vi "MoveAbs.vi"(8 "error in (no error)":errorcluster, 11 "ZanClass in":refnum<class "ZanClass.lvclass">) -> (0 "error out":errorcluster, 3 "ZanClass out":refnum<class "ZanClass.lvclass">)   [LabVIEW 2019, in "ZanClass.lvclass"]
uses:
  ZanClass.lvclass
  LLB/zmotion/zaux/zauxdll.lvlib
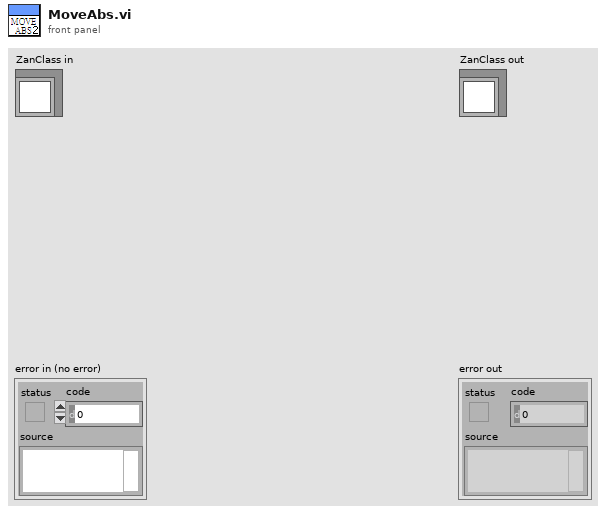
[diagram p1: front panel]
types:
  T1 = cluster{"AxisName":string, "Accel":dbl, "Deaccel":dbl, "Speed":dbl, "Sramp":dbl}[]
  T2 = typedef "IO Card_Type.ctl" = enum16{"None", "Unidaq32", "6480", "2410C-64", "Zan", "DMC1000B", "16InOut", "Robot", "DMC3600"}
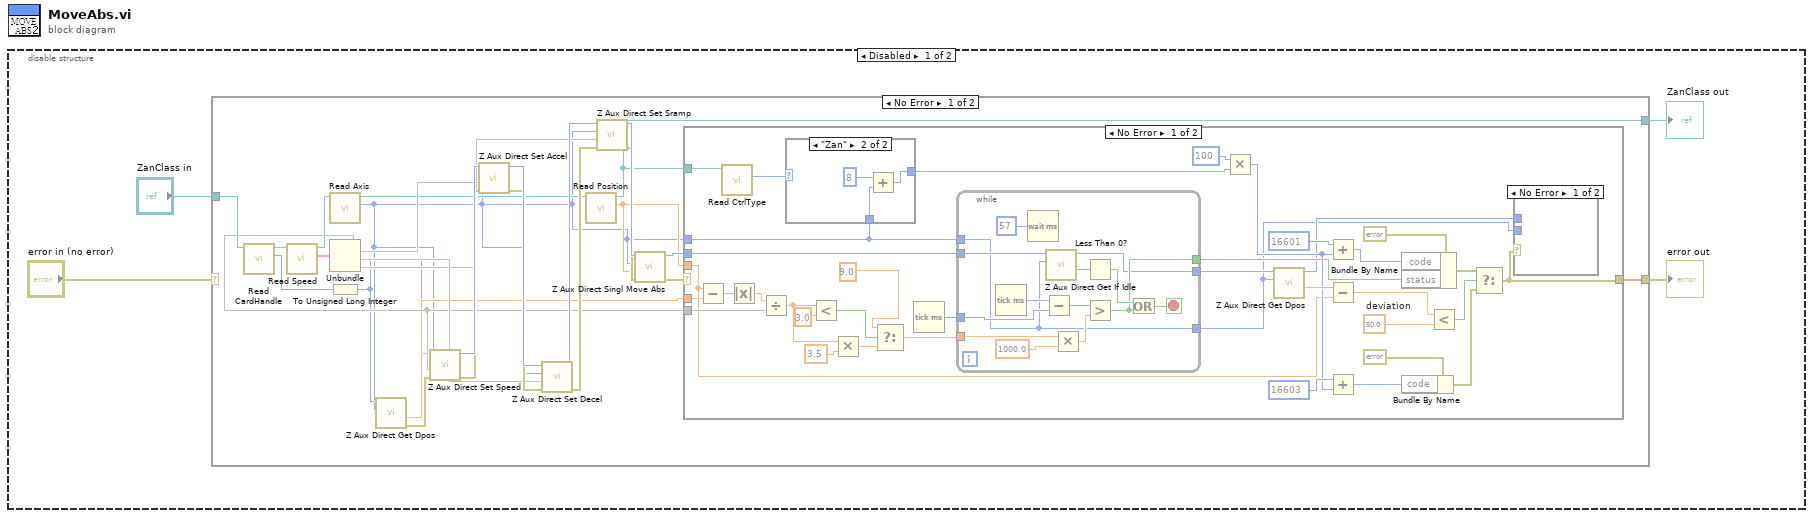
[diagram p0: block diagram]
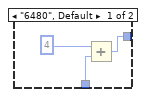
[diagram p2: hidden frame]
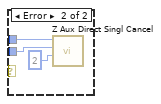
[diagram p3: hidden frame]
diagram:
  n1 = disable-structure shown="Disabled" {
    frame Disabled {
      n2 = case shown="No Error" "error in (no error)" {
        selector: "error in (no error)" -> [_ w93]
        tunnel: "ZanClass in" -> [w31 w94]
        tunnel: [w10 w93] -> w1
        tunnel: [w5 w94] -> w2
        frame No Error {
          n3 = call-dynamic "Read CardHandle.vi"("AxisCard in"=w31) -> ("CardHandle"=w30:i32, "AxisCard out"=w26:refnum<class "ZanClass.lvclass">)  [unwired: 8 in, 1 out]
          n4 = call-dynamic "Read Speed.vi"("AxisCard in"=w26) -> ("AxisSpeed"=w24:T1, "AxisCard out"=w25:refnum<class "ZanClass.lvclass">)  [unwired: 8 in, 1 out]
          n5 = call-dynamic "Read Axis.vi"("AxisCard in"=w25) -> ("Axis"=w6:u32, "AxisCard out"=w16:refnum<class "ZanClass.lvclass">)  [unwired: 8 in, 1 out]
          n6 = Unbundle(w24) -> (w12, w23, w19, w18)
          n7 = To Unsigned Long Integer(number=w30) -> (unsigned 32bit integer=w7:u32)
          n8 = call "Z Aux Direct Get Dpos.vi"("iaxis"=w6, "handle"=w7) -> ("error out"=w8:errorcluster, "pfValue out"=w9:sgl)  [unwired: 6 in, 2 out]
          n9 = call "Z Aux Direct Set Speed.vi"("error in (no error)"=w8, "fValue"=w12, "iaxis"=w6, "handle"=w7) -> ("error out"=w22:errorcluster, "handle out"=w29:u32)  [unwired: 5 in, 1 out]
          n10 = call "Z Aux Direct Set Accel.vi"("error in (no error)"=w22, "fValue"=w23, "iaxis"=w6, "handle"=w29) -> ("error out"=w21:errorcluster, "handle out"=w28:u32)  [unwired: 5 in, 1 out]
          n11 = call "Z Aux Direct Set Decel.vi"("error in (no error)"=w21, "fValue"=w19, "iaxis"=w6, "handle"=w28) -> ("error out"=w20:errorcluster, "handle out"=w27:u32)  [unwired: 5 in, 1 out]
          n12 = call-dynamic "Read Position.vi"("AxisCard in"=w16) -> ("Position"=w11:dbl, "AxisCard out"=w5:refnum<class "ZanClass.lvclass">)  [unwired: 8 in, 1 out]
          n13 = call "Z Aux Direct Set Sramp.vi"("error in (no error)"=w20, "fValue"=w18, "iaxis"=w6, "handle"=w27) -> ("error out"=w15:errorcluster, "handle out"=w17:u32)  [unwired: 5 in, 1 out]
          n14 = call "Z Aux Direct Singl Move Abs.vi"("error in (no error)"=w15, "fdistance"=w11, "iaxis"=w6, "handle"=w17) -> ("error out"=w14:errorcluster, "handle out"=w13:u32)  [unwired: 5 in, 1 out]
          n15 = case shown="No Error" w14 {
            selector: w14 -> [_ w92]
            tunnel: w13 -> [w68 _]
            tunnel: w6 -> [w35 _]
            tunnel: w12 -> [w46 _]
            tunnel: w11 -> [w40 _]
            tunnel: [w50 w92] -> w10
            tunnel: w9 -> [w39 _]
            tunnel: w5 -> [w38 _]
            frame No Error {
              w60 = 50.0  # deviation
              n16 = Subtract(x=w40, y=w39) -> (x-y=w42:dbl)
              n17 = call-dynamic "Read CtrlType.vi"("AxisCard in"=w38) -> ("IO Card Type"=w37:T2)  [unwired: 8 in, 2 out]
              n18 = Absolute Value(x=w42) -> (abs(x)=w41:dbl)
              n19 = Divide(x=w41, y=w46) -> (x/y=w33:dbl)
              n20 = case shown="\"Zan\"" w37 {
                tunnel: [w71 w74] -> w36
                tunnel: w35 -> [w69 w72]
                frame "6480", Default {
                  n21 = Add(x=4, y=w69) -> (x+y=w71:u32)
                }
                frame "Zan" {
                  n22 = Add(x=8, y=w72) -> (x+y=w74:u32)
                }
              }
              n23 = Less?(x=w33, y=3.0) -> (x < y?=w45:bool)
              n24 = Multiply(x=w33, y=3.5) -> (x*y=w44:dbl)
              n25 = Select(t=9.0, s=w45, f=w44) -> (s? t:f=w43:dbl)
              n26 = Tick Count (ms)() -> (millisecond timer value=w67:u32)
              n27 = while {
                tunnel: w68 -> [w91]
                tunnel: w35 -> [w79]
                tunnel: w67 -> [w86]
                tunnel: [w81] -> w54
                tunnel: [w80] -> w63
                tunnel: [w79] -> w48
                tunnel: w43 -> [w78]
                stop <- w82 stop-if-true
                n28 = Tick Count (ms)() -> (millisecond timer value=w87:u32)
                n29 = Wait (ms)(milliseconds to wait=u32 57) -> ()  [unwired: 1 out]
                n30 = Subtract(x=w87, y=w86) -> (x-y=w85:u32)
                n31 = call "Z Aux Direct Get If Idle.vi"("iaxis"=w79, "handle"=w91) -> ("piValue out"=w90:i32, "handle out"=w80:u32)  [unwired: 6 in, 2 out]
                n32 = Multiply(x=w78, y=1000.0) -> (x*y=w84:dbl)
                n33 = Less Than 0?(x=w90) -> (x < 0?=w83:bool)
                n34 = Greater?(x=w85, y=w84) -> (0:w81:bool)
                n35 = Or(x=w83, y=w81) -> (x .or. y?=w82:bool)
              }
              n36 = Multiply(x=u32 100, y=w36) -> (x*y=w58:u32)
              n37 = call "Z Aux Direct Get Dpos.vi"("iaxis"=w48, "handle"=w63) -> ("pfValue out"=w62:sgl, "handle out"=w49:u32)  [unwired: 6 in, 2 out]
              n38 = Add(x=16601 ("code"), y=w58) -> (x+y=w65:u32)
              n39 = Subtract(x=w62, y=w40) -> (x-y=w61:dbl)
              n40 = Add(x=16603 ("code"), y=w58) -> (x+y=w56:u32)
              n41 = Bundle By Name(cluster=errorcluster {"status"=FALSE, "code"=16601, "source"="MoveTimeOut"} ("error constant"), "code"=w65, "status"=w54) -> (w53:errorcluster)
              n42 = Bundle By Name(cluster=errorcluster {"status"=TRUE, "code"=16603, "source"="MovePosErr"} ("error constant"), "code"=w56) -> (w51:errorcluster)
              n43 = Less?(x=w61, y=w60) -> (x < y?=w55:bool)
              n44 = Select(t=w53, s=w55, f=w51) -> (s? t:f=w50:errorcluster)
              n45 = case shown="No Error" w50 {
                tunnel: w49 -> [_ w77]
                tunnel: w48 -> [_ w76]
                frame No Error {
                }
                frame Error {
                  n46 = call "Z Aux Direct Singl Cancel.vi"("imode"=2, "iaxis"=w76, "handle"=w77) -> ()  [unwired: 6 in, 3 out]
                }
              }
            }
            frame Error {
            }
          }
        }
        frame Error {
        }
      }
      "error out" <- w1
      "ZanClass out" <- w2
    }
    frame Enabled {
    }
  }
